vi "创建鹰对象.vi"() -> (3 "eagle.lvclass":refnum<class "eagle.lvclass">)   [LabVIEW 2020, in "eagle.lvclass"]
uses:
  eagle.lvclass
  Animal/Animal.lvclass/Animal.ctl
  Animal/Animal.lvclass
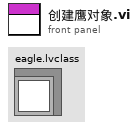
[diagram p1: front panel]
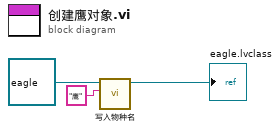
[diagram p0: block diagram]
diagram:
  n1 = call "写入物种名.vi"("物种名"="鹰", "Animal输入"=refnum<class "eagle.lvclass"> refnum ("eagle.lvclass")) -> ("Animal输出"=→"eagle.lvclass":refnum<class "eagle.lvclass">)  [unwired: 8 in, 1 out]
